vi "Waveform Buffer Generation-Current (multi).vi"(0 "task/channels in":refnum<k21>, 1 "Samples per Buffer":dbl=1000.0, 3 "Amplitude":dbl=2.0 format="%0.2p", 5 "Desired Frequency":dbl=1000.0 format="%.2f", 7 "Offset":dbl=0.01 format="%0.2p", 9 "Waveform Type":T1(ring), 11 "error in (no error)":errorcluster, 12 "Cycles per Buffer":dbl=1.0 format="%.2f") -> (4 "task out":refnum<k21>, 6 "Waveform":waveform(dbl)[](array[waveform]), 10 "Resulting Frequency":dbl format="%.2f", 14 "Resulting Sample Clock Rate":dbl format="%.2f", 15 "error out":errorcluster)   [LabVIEW 2010]
doc: "This subVI is used to create a Sine, Square, Triangle or Sawtooth Waveform. The inputs to this VI are the Waveform Type, which determines if the output waveform is a Sine, Square, Triangle, or Sawtooth Waveform, the amplitude, Desired Frequency, Samples per Buffer, and Cycles per Buffer. \n\nThe Desired Frequency, Samples per Buffer, and Cycles per Buffer are used to calculate the sample clock rate. The DAQmx Timing property node sets the sample clock rate for the device specified in the task/channels in control. \n\nThe actual, coerced, sample clock rate is returned and used as an input to the Basic Function Generator.vi. The Basic Function Generator returns a waveform of data with timing information.\n\nThe formula below was used to determine the sample clock rate:\n\nDesired Frequency=[(Cycles/Buffer)X(Sample Clock Rate)]/Samples per Buffer\n\nNote: The Block Diagram rearranges the variables to solve for Sample Clock Rate"
uses:
  <vilib>/measure/NI_MABase.lvlib
  D:/ProgramFiles/National Instruments/LabVIEW 2010/resource/objmgr/daqmx.rc
panel:
  out "Samples/cycle":dbl format="%0.2f"
  out "Desired Sample Clock Rate":dbl format="%.2f"
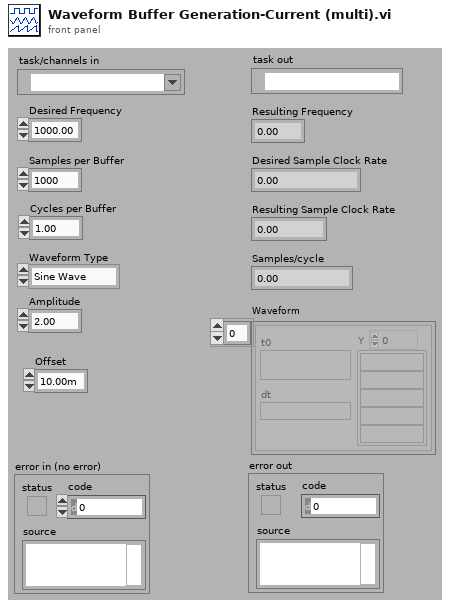
[diagram p1: front panel]
types:
  T1 = enum16{"Sine Wave", "Triangle Wave", "Square Wave", "Sawtooth Wave"}
  T2 = cluster{"SampClk.Rate":dbl, "Samples per Buffer":dbl}
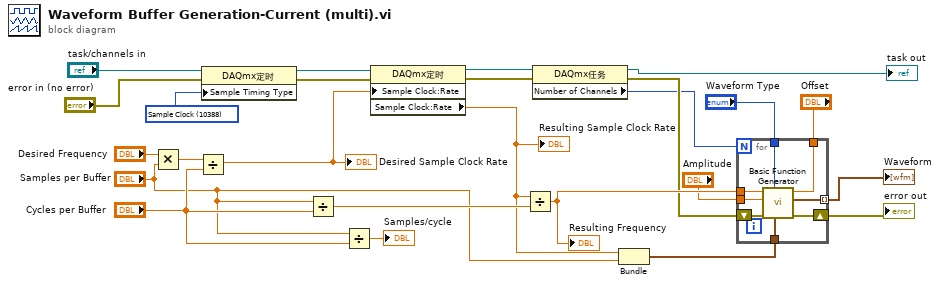
[diagram p0: block diagram]
diagram:
  w10 = 10388 items=["Sample Clock"=10388, "Handshake"=10389, "Implicit"=10451, "On Demand"=10390, "Change Detection"=12504] ("SampTimingType")
  n1 = Multiply(x="Desired Frequency", y="Samples per Buffer") -> (x*y=w22:dbl)
  n2 = Divide(x=w22, y="Cycles per Buffer") -> (x/y=w18:dbl)
  "Desired Sample Clock Rate" <- w18
  n3 = property class="DAQmx定时"(reference="task/channels in", error in="error in (no error)", "Sample Timing Type"=w10) -> (reference out=w12:refnum<k21>, error out=w11:errorcluster)
  n4 = Divide(x="Samples per Buffer", y="Cycles per Buffer") -> (x/y=w19:dbl)
  n5 = Divide(x="Samples per Buffer", y="Cycles per Buffer") -> (x/y=→"Samples/cycle":dbl)
  n6 = property class="DAQmx定时"(reference=w12, error in=w11, "Sample Clock:Rate"=w18) -> (reference out=w6:refnum<k21>, error out=w5:errorcluster, "Sample Clock:Rate"=w14:dbl)
  "Resulting Sample Clock Rate" <- w14
  n7 = Divide(x=w14, y=w19) -> (x/y=w25:dbl)
  "Resulting Frequency" <- w25
  n8 = property class="DAQmx任务"(reference=w6, error in=w5) -> (reference out=→"task out":refnum<k21>, error out=w4:errorcluster, "Number of Channels"=w2:u32)
  n9 = Bundle("SampClk.Rate"=w14, "Samples per Buffer"="Samples per Buffer") -> (w23:T2)  [unwired: 1 in]
  n10 = for {
    N: w2 -> [_]
    tunnel: w25 -> [w33]
    tunnel: w23 -> [w32]
    tunnel: [w31] -> w1 mode=indexing
    tunnel: "Waveform Type" -> [w30]
    tunnel: "Amplitude" -> [w29]
    tunnel: "Offset" -> [w27]
    shift-right: [w28] -> w13
    shift-left: w4 -> [w26]
    n11 = call <vilib>:"Basic Function Generator.vi"("offset"=w27, "sampling info"=w32, "signal type"=w30, "error in (no error)"=w26, "amplitude"=w29, "frequency"=w33) -> ("error out"=w28:errorcluster, "signal out"=w31:waveform(dbl))  [unwired: 3 in, 1 out]
  }
  "error out" <- w13
  "Waveform" <- w1
